vi "List.vi"(8 "error in (no error)":errorcluster) -> (0 "error out":errorcluster, 3 "COM ports":string[](array[string]))   [LabVIEW 2011, in "Thorlabs_MDT69xB.lvlib"]
uses:
  <instrlib>/Thorlabs_MDT69xB/Thorlabs_MDT69xB.lvlib
  <instrlib>/Thorlabs_MDT69xB/Data/MDT_COMMAND_LIB_win32.dll
  <instrlib>/Thorlabs_MDT69xB/Data/MDT_COMMAND_LIB_x64.dll
panel:
  out "Serial Number":u8[](array[numeric])
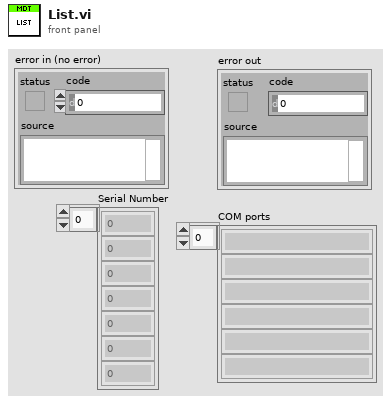
[diagram p1: front panel]
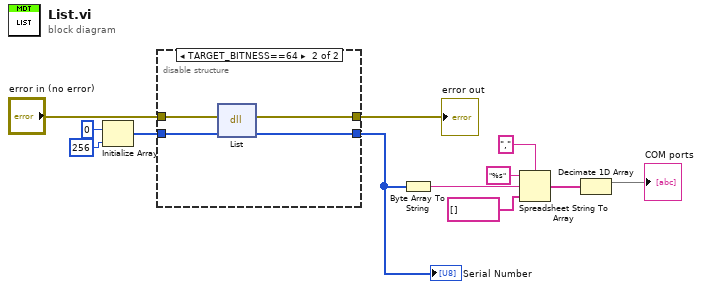
[diagram p0: block diagram]
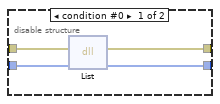
[diagram p2: hidden frame]
diagram:
  n1 = Initialize Array(u8 0 ("element"), 256 ("dimension size")) -> (w12:u8[])
  n2 = disable-structure shown="TARGET_BITNESS==64" {
    disable-tunnel: w12 -> [w16 w20]
    disable-tunnel: "error in (no error)" -> [w15 w19]
    disable-tunnel: [w14 w18] -> w8
    disable-tunnel: [w13 w17] -> w7
    frame condition #0 {
      n3 = dll-call lib="C:/Program Files (x86)/National Instruments/LabVIEW 2011/instr.lib/Thorlabs_MDT69xB/Data/MDT_COMMAND_LIB_win32.dll" fn="List"(error in=w15, "Serial Number"=w16) -> (error out=w13:errorcluster, "Serial Number"=w14:u8[])  [unwired: 3 in, 1 out]
    }
    frame condition #1 (active) {
      n4 = dll-call lib="C:/Program Files/National Instruments/LabVIEW 2011/instr.lib/Thorlabs_MDT69xB/Data/MDT_COMMAND_LIB_x64.dll" fn="List"(error in=w19, "Serial Number"=w20) -> (error out=w17:errorcluster, "Serial Number"=w18:u8[])  [unwired: 3 in, 1 out]
    }
  }
  "error out" <- w7
  "Serial Number" <- w8
  n5 = Byte Array To String(unsigned byte array=w8) -> (string=w5:string)
  n6 = Spreadsheet String To Array(delimiter (Tab)=",", format string="%s", spreadsheet string=w5, array type (2D Dbl)=string[] []) -> (array=w2:string[])
  n7 = Decimate 1D Array(w2) -> (→"COM ports":string[])  [unwired: 1 out]
